vi "Configure IQ Adjustment.vi"(0 "VISA resource name":refnum<visa-resource-name>, 1 "I Offset (0 percent)":dbl, 2 "Enable I/Q Adjustment (F:Disable)":bool, 5 "Q Offset (0 percent)":dbl, 7 "Gain (0 dB)":dbl, 9 "Quadrature Skew (0 deg)":dbl, 11 "error in (no error)":errorcluster, 12 "I/Q Skew (0 s)":dbl, 13 "I/Q Timing Skew Path (0: RF)":u16(ring) items=["RF", "Baseband"], 14 "I/Q Delay (0 s)":dbl) -> (4 "VISA resource name out":refnum<visa-resource-name>, 15 "error out":errorcluster)   [LabVIEW 2011, in "Agilent PSG MXG Series.lvlib"]
doc: "Configures I/Q adjustments.\n\n<B>Notes:</B>\n(1) This VI is valid only in E8267C, E8267D, N5182A.\n\n(2) For E8267C, this VI is valid only when the instrument installs <B>Option 002</B> (Internal baseband generator) or <B>Option 602</B> (Digital bus baseband generator)."
uses:
  Agilent PSG MXG Series.lvlib
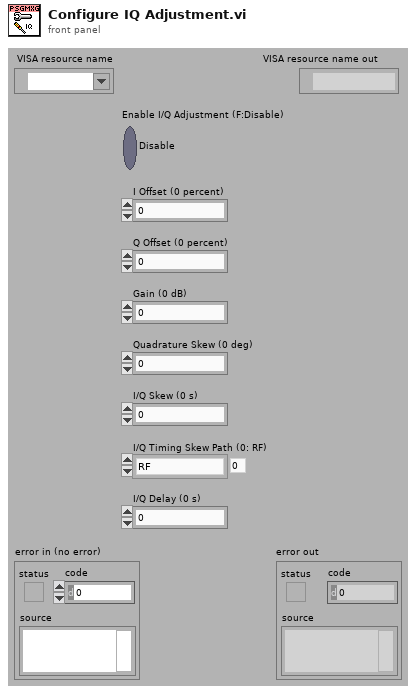
[diagram p1: front panel]
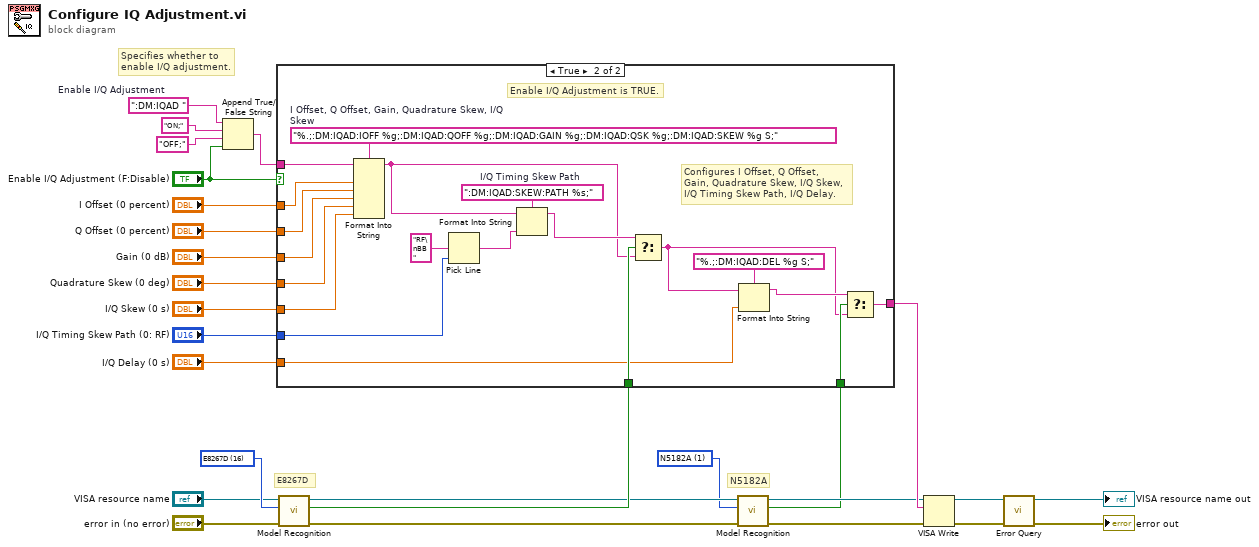
[diagram p0: block diagram]
diagram:
  w8 = u16 1 items=["N5181A"=0, "N5182A"=1, "E8241A"=5, "E8244A"=6, "E8251A"=7, "E8254A"=8, "E8247C"=10, "E8257C"=11, "E8267C"=12, "E8257D"=15, "E8267D"=16] ("Model Type (0: N5181A)")
  w12 = u16 16 items=["N5181A"=0, "N5182A"=1, "E8241A"=5, "E8244A"=6, "E8251A"=7, "E8254A"=8, "E8247C"=10, "E8257C"=11, "E8267C"=12, "E8257D"=15, "E8267D"=16] ("Model Type (0: N5181A)")
  w27 = ":DM:IQAD "  # Enable I/Q Adjustment
  # "Specifies whether to\nenable I/Q adjustment."
  # "E8267D"
  # "N5182A"
  n1 = Append True/False String(1:"Enable I/Q Adjustment (F:Disable)", 2:"OFF;" ("false string"), 3:"ON;" ("true string"), 4:w27) -> (0:w23:string)
  n2 = call "Model Recognition.vi"("error in (no error)"="error in (no error)", "Model Type (0: N5181A)"=w12, "VISA resource name"="VISA resource name") -> ("error out"=w9:errorcluster, "Is Model Correct"=w11:bool, "VISA resource name out"=w10:refnum<visa-resource-name>)  [unwired: 6 in]
  n3 = call "Model Recognition.vi"("error in (no error)"=w9, "Model Type (0: N5181A)"=w8, "VISA resource name"=w10) -> ("error out"=w6:errorcluster, "Is Model Correct"=w5:bool, "VISA resource name out"=w7:refnum<visa-resource-name>)  [unwired: 6 in]
  n4 = case shown="True" "Enable I/Q Adjustment (F:Disable)" {
    tunnel: w23 -> [w28 w47]
    tunnel: "I Offset (0 percent)" -> [_ w46]
    tunnel: "Q Offset (0 percent)" -> [_ w45]
    tunnel: "Gain (0 dB)" -> [_ w44]
    tunnel: "Quadrature Skew (0 deg)" -> [_ w43]
    tunnel: "I/Q Skew (0 s)" -> [_ w42]
    tunnel: "I/Q Timing Skew Path (0: RF)" -> [_ w40]
    tunnel: w11 -> [_ w37]
    tunnel: "I/Q Delay (0 s)" -> [_ w33]
    tunnel: w5 -> [_ w32]
    tunnel: [w28 w29] -> w15
    frame False {
      # "Enable I/Q Adjustment is FALSE."
    }
    frame True {
      w39 = ":DM:IQAD:SKEW:PATH %s;"  # I/Q Timing Skew Path
      w48 = "%.;:DM:IQAD:IOFF %g;:DM:IQAD:QOFF %g;:DM:IQAD:GAIN %g;:DM:IQAD:QSK %g;:DM:IQAD:SKEW %g S;"  # I Offset, Q Offset, Gain, Quadrature Skew, I/Q Skew
      # "Configures I Offset, Q Offset,\nGain, Quadrature Skew, I/Q Skew,\nI/Q Timing Skew Path, I/Q Delay."
      # "Enable I/Q Adjustment is TRUE."
      n5 = Format Into String(format string=w48, initial string=w47, w46, w45, w44, w43, w42) -> (resulting string=w35:string)  [unwired: 1 in, 1 out]
      n6 = Pick Line(multi-line string="RF\nBB", line index=w40) -> (output string=w38:string)  [unwired: 1 in]
      n7 = Format Into String(format string=w39, initial string=w35, w38) -> (resulting string=w36:string)  [unwired: 1 in, 1 out]
      n8 = Select(t=w36, s=w37, f=w35) -> (s? t:f=w30:string)
      n9 = Format Into String(format string="%.;:DM:IQAD:DEL %g S;", initial string=w30, w33) -> (resulting string=w31:string)  [unwired: 1 in, 1 out]
      n10 = Select(t=w31, s=w32, f=w30) -> (s? t:f=w29:string)
    }
  }
  n11 = VISA Write(VISA resource name=w7, write buffer=w15, error in (no error)=w6) -> (VISA resource name out=w14:refnum<visa-resource-name>, error out=w13:errorcluster)  [unwired: 1 out]
  n12 = call "Error Query.vi"("error in (no error)"=w13, "VISA resource name"=w14) -> ("error out"=→"error out":errorcluster, "VISA resource name out"=→"VISA resource name out":refnum<visa-resource-name>)  [unwired: 6 in, 2 out]
